vi "test_ShowUI.vi"(8 "error in (no error)":errorcluster, 11 "TestCase in":refnum<class "SMO.UI_TestCase.lvclass">) -> (0 "error out":errorcluster, 3 "TestCase out":refnum<class "SMO.UI_TestCase.lvclass">)   [LabVIEW 2013, in "SMO.UI_TestCase.lvclass"]
uses:
  SMO.UI_TestCase.lvclass
  SMO.UI_TestCase.lvclass/SMO.UI_TestCase.ctl
  <vilib>/addons/_JKI Toolkits/VI Tester/TestCase.llb/TestCase.lvclass
  src/SMO.UI/SMO.UI.lvclass
  src/SMO/SMO.lvclass
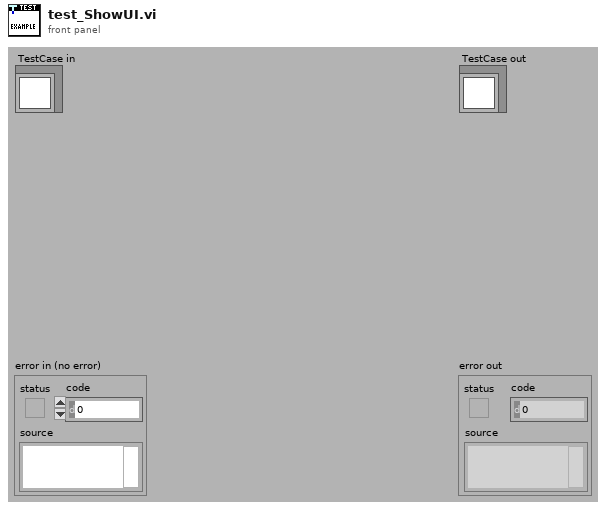
[diagram p1: front panel]
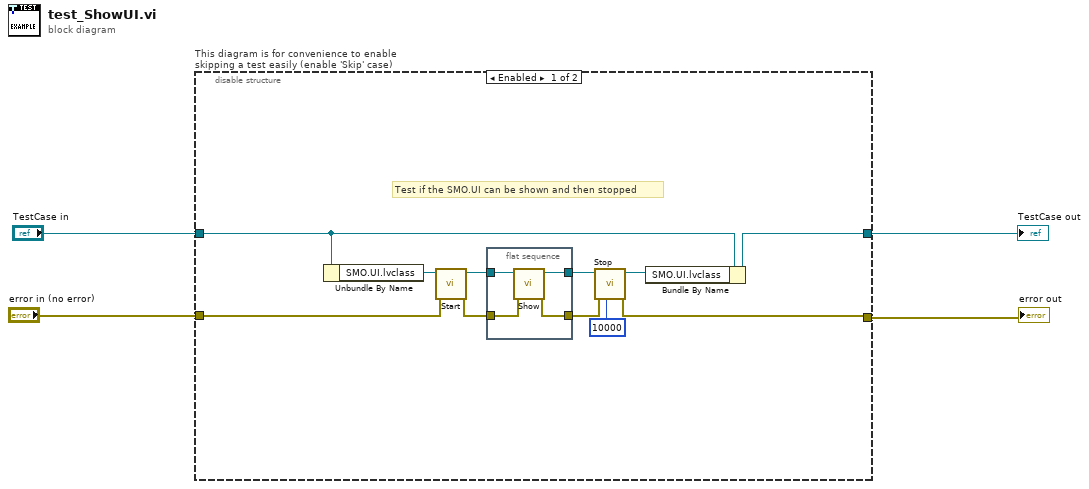
[diagram p0: block diagram]
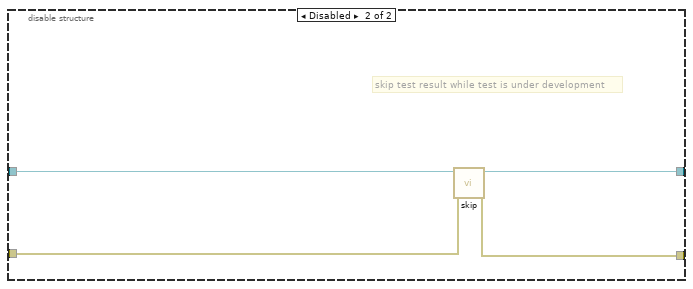
[diagram p2: hidden frame]
diagram:
  n1 = disable-structure "This diagram is for convenience to enable skipping a test easily (enable 'Skip' case)" shown="Enabled" {
    disable-tunnel: "TestCase in" -> [w15 w23]
    disable-tunnel: [w14 w21] -> w1
    disable-tunnel: [w6 w22] -> w3
    disable-tunnel: "error in (no error)" -> [w11 w20]
    frame Enabled {
      # "Test if the SMO.UI can be shown and then stopped"
      n2 = Unbundle By Name(w15) -> ("SMO.UI.lvclass"=w13:refnum<class "SMO.UI.lvclass">)
      n3 = call "Start.vi"("error in (no error)"=w11, "SMO"=w13) -> ("error out"=w10:errorcluster, "SMO out"=w12:refnum<class "SMO.UI.lvclass">)  [unwired: 8 in]
      n4 = flat-sequence {
        tunnel: w12 -> [w19]
        tunnel: w10 -> [w18]
        tunnel: [w17] -> w9
        tunnel: [w16] -> w7
        frame #0 {
          n5 = call "Show.vi"("error in (no error)"=w18, "SMO.UI"=w19) -> ("error out"=w16:errorcluster, "SMO.UI out"=w17:refnum<class "SMO.UI.lvclass">)  [unwired: 8 in]
        }
      }
      n6 = call "Stop.vi"("timeout in ms (-1)"=10000, "error in (no error)"=w7, "SMO"=w9) -> ("error out"=w6:errorcluster, "SMO out"=w8:refnum<class "SMO.UI.lvclass">)  [unwired: 7 in]
      n7 = Bundle By Name(cluster=w15, "SMO.UI.lvclass"=w8) -> (w14:refnum<class "SMO.UI_TestCase.lvclass">)
    }
    frame Disabled {
      # "skip test result while test is under development"
      n8 = call <vilib>:"skip.vi"("error in (no error)"=w20, "TestCase in"=w23) -> ("error out"=w22:errorcluster, "TestCase out"=w21:refnum<class "SMO.UI_TestCase.lvclass">)  [unwired: 8 in]
    }
  }
  "error out" <- w3
  "TestCase out" <- w1
